vi "LVLibNameFromFilePath.vi"(8 "error in (no error)":errorcluster, 11 "LV File Path":path) -> (0 "error out":errorcluster, 3 "Library / Class Name":string)   [LabVIEW 2019, in "Hawkeye.lvlib"]
uses:
  Hawkeye.lvlib
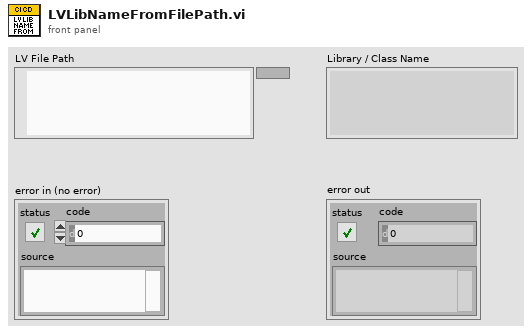
[diagram p1: front panel]
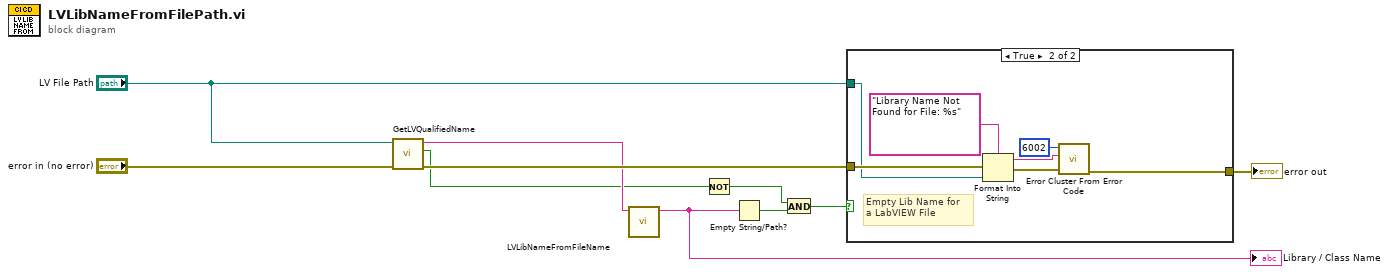
[diagram p0: block diagram]
diagram:
  n1 = call "GetLVQualifiedName.vi"("error in (no error)"="error in (no error)", "LV File Path"="LV File Path") -> ("error out"=w3:errorcluster, "Non LabVIEW File?"=w1:bool, "VI Name / CTL Name / LVCLASS Name"=w2:string)  [unwired: 7 in]
  n2 = call "LVLibNameFromFileName.vi"("VI Name / CTL Name / LVCLASS Name"=w2) -> ("Library Name"=w10:string)  [unwired: 10 in]
  "Library / Class Name" <- w10
  n3 = Not(x=w1) -> (.not. x?=w7:bool)
  n4 = Empty String/Path?(string/path=w10) -> (empty?=w8:bool)
  n5 = And(x=w7, y=w8) -> (x .and. y?=w6:bool)
  n6 = case shown="True" w6 {
    tunnel: w3 -> [w11 w18]
    tunnel: "LV File Path" -> [_ w14]
    tunnel: [w11 w12] -> w9
    frame False {
    }
    frame True {
      # "Empty Lib Name for\na LabVIEW File"
      n7 = Format Into String(format string="Library Name Not Found for File: %s", error in=w18, w14) -> (resulting string=w13:string, error out=w17:errorcluster)  [unwired: 1 in]
      n8 = call <vilib>:"Error Cluster From Error Code.vi"("error in (no error)"=w17, "error message (\"\")"=w13, "error code (0)"=6002) -> ("error out"=w12:errorcluster)  [unwired: 6 in]
    }
  }
  "error out" <- w9
